vi "OriginalTemplate.vi"() -> ()   [LabVIEW 2017]
uses:
  <vilib>/rvi/Emulation/niFpgaGetClockAttributes.vi
  <vilib>/rvi/Emulation/niFpgaSctlEmulationGetInTimedLoop.vi
  <vilib>/rvi/Emulation/niFpgaEmulationReportErrorSimple.vi
  <vilib>/rvi/Emulation/niFpgaProcessEmulError.vi
  <vilib>/rvi/interface/RandomDataEmulation/niFpgaRandomDataHandleErrors.vi
  <vilib>/rvi/Emulation/niFpgaCriticalErrorInLSC.vi
  <vilib>/rvi/DataTransferAndStorage/Container/XNode/niFpgaContainer.xnode
  <vilib>/rvi/interface/RandomDataEmulation/nirviRandomDataFpgaReadWriteTemplate.vi
panel:
  out "FPGA Error":errorcluster
  out "Finished":bool
  in  "stop":bool
  out "Module Underflow":bool
  out "Acq Loop Ticks":u32
  out "DMA FIFO Full":bool
  out "Chan Count":bool
  out "First Read":bool
  in  "Number of Channels":i32=4
  in  "Acquisition Type":enum16{"Finite Samples", "Continuous Samples"}(ring)
  in  "Samps per Chan [Finite]":i32=5120
  out "oclk mult":u32
  out "oclk div":u32
  out "oclk freq":u32
  in  "data rate (S/s)":u32
  # "Total Slices: 27.5% (3663 out of 13300)\nSlice Registers: 9.3% (9885 out of 106400)\nSlice LUTs: 18.3% (9725 out of 53200)\nBlock RAMs: 5.0% (7 out of 140)\nDSP48s: 0.0% (0 out of 220)"
  # "Array size fixed at 40\nelements but may be \nexpanded if needed"
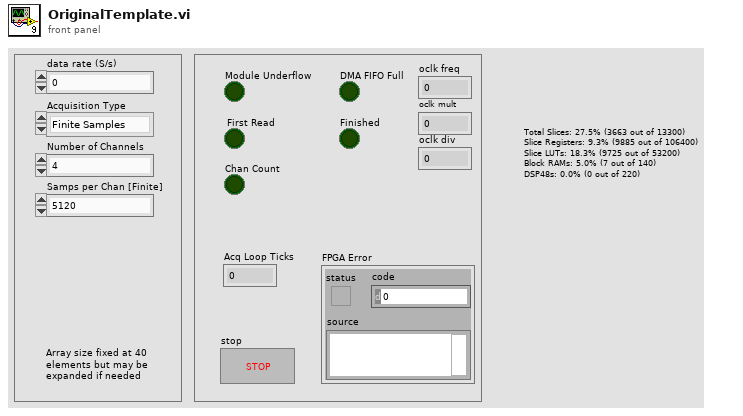
[diagram p1: front panel]
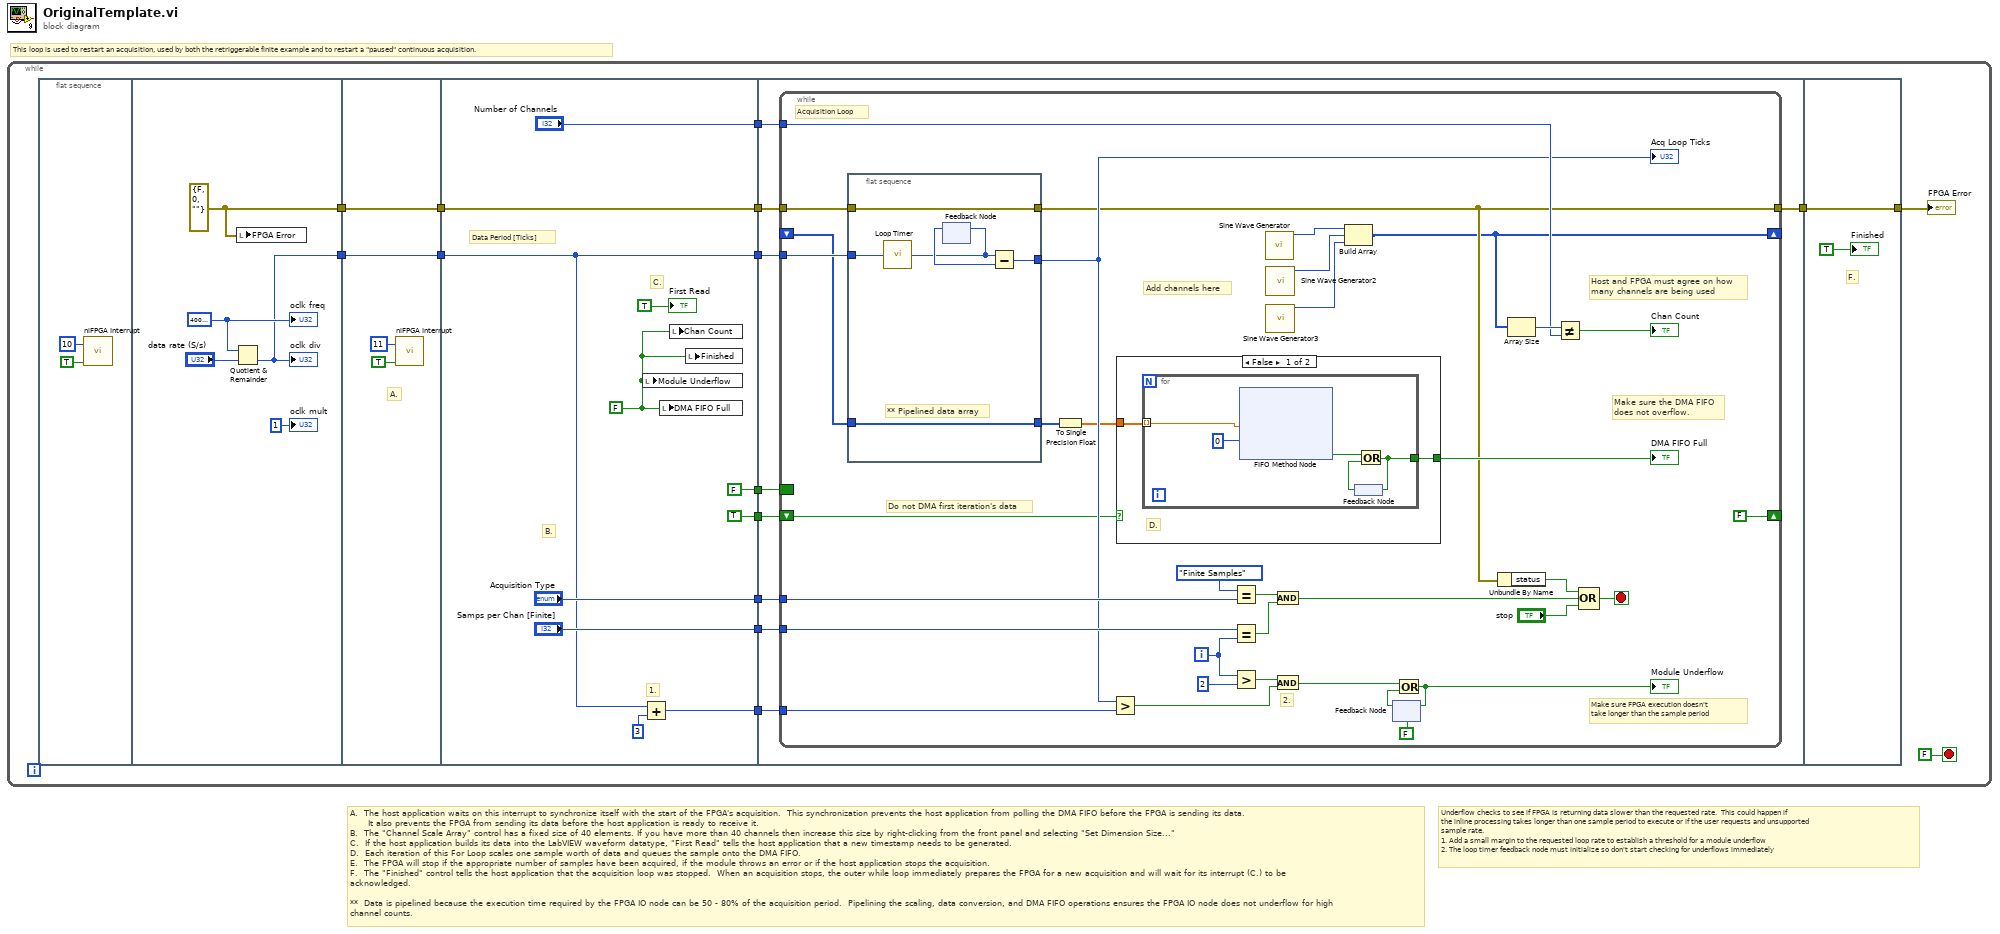
[diagram p0: block diagram]
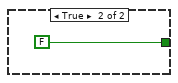
[diagram p2: hidden frame]
diagram:
  # "Underflow checks to see if FPGA is returning data slower than the requested rate.  This could happen if\nthe inline processing takes longer than one sample period to execute or if the user requests and unsupported\nsample rate.\n1. Add a small margin to the requested loop rate to establish a threshold for a module underflow \n2. The loop timer feedback node must initialize so don't start checking for underflows immediately"
  # "A.  The host application waits on this interrupt to synchronize itself with the start of the FPGA's acquisition.  This synchronization prevents the host application from polling the DMA FIFO before the FPGA is sending its data.\n      It also prevents the FPGA from sending its data before the host application is ready to receive it.\nB.  The \"Channel Scale Array\" control has a fixed size of 40 elements. If you have more than 40 channels then increase this size by right-clicking from the front panel and selecting \"Set Dimension Size...\"\nC.  If the host application builds its data into the LabVIEW waveform datatype, \"First Read\" tells the host application that a new timestamp needs to be generated.\nD.  Each iteration of this For Loop scales one sample worth of data and queues the sample onto the DMA FIFO.  \nE.  The FPGA will stop if the appropriate number of samples have been acquired, if the module throws an error or if the host application stops the acquisition.  \nF.  The \"Finished\" control tells the host application that the acquisition loop was stopped.  When an acquisition stops, the outer while loop immediately prepares the FPGA for a new acquisition and will wait for its interrupt (C.) to be acknowledged. \n\n**  Data is pipelined because the execution time required by the FPGA IO node can be 50 - 80% of the acquisition period.  Pipelining the scaling, data conversion, and DMA FIFO operations ensures the FPGA IO node does not underflow for high\nchannel counts."
  # "This loop is used to restart an acquisition, used by both the retriggerable finite example and to restart a \"paused\" continuous acquisition."
  n1 = while {
    stop <- FALSE stop-if-true
    n2 = flat-sequence {
      tunnel: [w19] -> w7
      tunnel: [w18] -> w3
      tunnel: w7 -> [w24]
      tunnel: [w24] -> w6
      tunnel: [w23] -> w4
      tunnel: w3 -> [w23]
      tunnel: ["Number of Channels"] -> w15
      tunnel: ["Acquisition Type"] -> w14
      tunnel: ["Samps per Chan [Finite]"] -> w13
      tunnel: [w28] -> w12
      tunnel: [w31] -> w11
      tunnel: [TRUE] -> w10
      tunnel: w6 -> [w29]
      tunnel: [w29] -> w5
      tunnel: w4 -> [w28]
      tunnel: [FALSE] -> w2
      tunnel: w15 -> [w46]
      tunnel: w14 -> [w43]
      tunnel: w13 -> [w42]
      tunnel: w12 -> [w44]
      tunnel: w11 -> [w41]
      tunnel: w10 -> [w40]
      tunnel: [w39] -> w8
      tunnel: w5 -> [w45]
      tunnel: w2 -> [w38]
      tunnel: [w96] -> w9
      tunnel: w8 -> [w96]
      frame #0 {
        n3 = call <vilib>:"niFPGA Interrupt.vi"("Wait Until Cleared (F)"=TRUE ("Wait Until Cleared"), "IRQ Number (0)"=u8 10 ("IRQ Number")) -> ()  [unwired: 1 in]
      }
      frame #1 {
        w19 = errorcluster {"status"=FALSE, "code"=0, "source"=""} ("FPGA Error")
        w20 = u32 40000000 ("oclk freq")
        n4 = Quotient & Remainder(x=w20, y="data rate (S/s)") -> (floor(x/y)=w18:u32)  [unwired: 1 out]
        "oclk div" <- w18
        n5 = local write "FPGA Error"(w19) -> ()
        "oclk mult" <- u32 1 ("oclk mult")
        "oclk freq" <- w20
      }
      frame #2 {
        # "A."
        n6 = call <vilib>:"niFPGA Interrupt.vi"("Wait Until Cleared (F)"=TRUE ("Wait Until Cleared"), "IRQ Number (0)"=u8 11 ("IRQ Number")) -> ()  [unwired: 1 in]
      }
      frame #3 {
        w36 = FALSE ("Module Underflow")
        # "Data Period [Ticks]"
        # "1."
        # "C."
        # "B."
        n7 = Add(x=w28, y=u32 3) -> (x+y=w31:u32)
        n8 = local write "Module Underflow"(w36) -> ()
        n9 = local write "DMA FIFO Full"(w36) -> ()
        n10 = local write "Chan Count"(w36) -> ()
        n11 = local write "Finished"(w36) -> ()
        "First Read" <- TRUE ("First Read")
      }
      frame #4 {
        n12 = while {
          tunnel: w43 -> [w74]
          tunnel: w42 -> [w73]
          shift-right: [w47] -> _
          shift-left: _ -> [w65]
          tunnel: w46 -> [w75]
          tunnel: w45 -> [w67]
          tunnel: [w51] -> w39
          tunnel: w44 -> [w72]
          tunnel: w41 -> [w68]
          shift-right: [FALSE] -> _
          shift-left: w40 -> [w64]
          border: w38 -> [_]
          i -> [w62]
          stop <- w79 stop-if-true
          # "Add channels here"
          # "2."
          # "Do not DMA first iteration's data"
          # "Host and FPGA must agree on how \nmany channels are being used"
          # "Acquisition Loop"
          # "Make sure the DMA FIFO\ndoes not overflow."
          # "Make sure FPGA execution doesn't\ntake longer than the sample period"
          n13 = flat-sequence {
            tunnel: w72 -> [w94]
            tunnel: [w95] -> w51
            tunnel: w67 -> [w95]
            tunnel: [w91] -> w66
            tunnel: [w90] -> w53
            tunnel: w65 -> [w90]
            frame #0 {
              # "** Pipelined data array"
              n14 = call "Loop Timer"("Count(Ticks)"=w94) -> ("Tick Count(Ticks)"=w92:u32)
              n15 = feedback-in #1(w92) -> ()
              n16 = feedback #1() -> (w93:u32)  [unwired: 1 out]
              n17 = Subtract(x=w92, y=w93) -> (x-y=w91:u32)
            }
          }
          n18 = To Single Precision Float(number=w53) -> (single precision float=w52:sgl[])
          n19 = Greater?(x=w66, y=w68) -> (0:w71:bool)
          n20 = case shown="False" w64 {
            tunnel: [w83 FALSE] -> w78
            tunnel: w52 -> [w82 _]
            frame False {
              # "D."
              n21 = for {
                tunnel: [w87] -> w83
                tunnel: w82 -> [w85] mode=indexing
                n22 = xnode ("FIFO Method Node")("Element"=w85, "Timeout"=0) -> ("Timed Out?"=w86:bool)  [unwired: 1 in, 1 out]
                n23 = feedback #2() -> (w88:bool)
                n24 = Or(x=w86, y=w88) -> (x .or. y?=w87:bool)
                n25 = feedback-in #2(w87) -> ()
              }
            }
            frame True {
            }
          }
          "DMA FIFO Full" <- w78
          n26 = Equal?(x=enum16{"Finite Samples", "Continuous Samples"}."Finite Samples" ("y"), y=w74) -> (x = y?=w56:bool)
          n27 = Equal?(x=w73, y=w62) -> (x = y?=w55:bool)
          n28 = Greater?(x=w62, y=2) -> (0:w70:bool)
          n29 = call "Sine Wave Generator"() -> ("sine out"=w50:i16)  [unwired: 15 in]
          n30 = call "Sine Wave Generator2"() -> ("sine out"=w49:i16)  [unwired: 15 in]
          n31 = call "Sine Wave Generator3"() -> ("sine out"=w48:i16)  [unwired: 15 in]
          n32 = And(x=w56, y=w55) -> (x .and. y?=w54:bool)
          n33 = And(x=w70, y=w71) -> (x .and. y?=w58:bool)
          n34 = Build Array(w50, w49, w48) -> (w47:i16[])
          n35 = feedback #3(FALSE) -> (w60:bool)
          n36 = Or(x=w58, y=w60) -> (x .or. y?=w57:bool)
          "Module Underflow" <- w57
          n37 = feedback-in #3(w57) -> ()
          n38 = Unbundle By Name(w51) -> ("status"=w61:bool)
          n39 = Array Size(array=w47) -> (size(s)=w77:i32)
          n40 = Not Equal?(x=w77, y=w75) -> (x != y?=→"Chan Count":bool)
          n41 = Compound Arithmetic op=OR(w61, w54, "stop") -> (w79:bool)
          "Acq Loop Ticks" <- w66
        }
      }
      frame #5 {
        # "F."
        "Finished" <- TRUE ("Finished")
      }
    }
    "FPGA Error" <- w9
  }
